vi "ExtractScleraPlane.vi"(11 "Image In":T1) -> (3 "Image Out":T1)   [LabVIEW 2014]
uses:
  <vilib>/vision/Image Controls.llb/IMAQ Image.ctl
  <vilib>/vision/NI_Vision_Development_Module.lvlib
panel:
  out "error out":errorcluster
  in  "error in":errorcluster
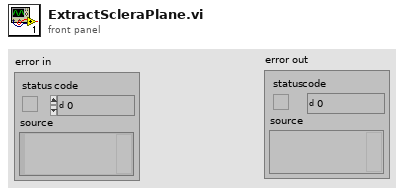
[diagram p1: front panel]
types:
  T1 = typedef "IMAQ Image.ctl" = refnum<image>
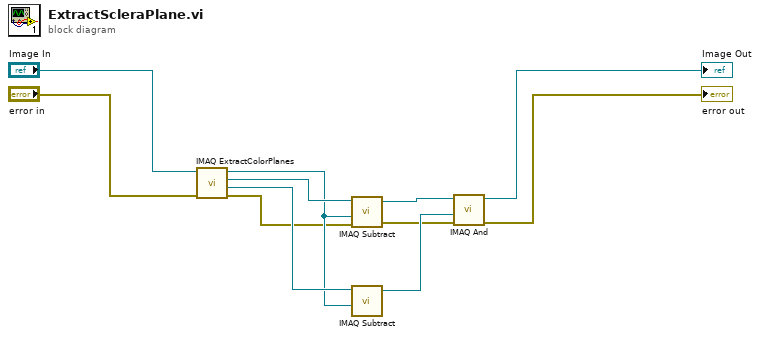
[diagram p0: block diagram]
diagram:
  n1 = call "IMAQ ExtractColorPlanes"("error in (no error)"="error in", "Image Src"="Image In") -> ("error out"=w3:errorcluster, "Blue or Luma or Val or Inten Plane out"=w8:T1, "Green or Sat Plane out"=w9:T1, "Red or Hue Plane out"=w7:T1)  [unwired: 6 in]
  n2 = call "IMAQ Subtract"("Image Src A"=w9, "Image Src B"=w7, "error in (no error)"=w3) -> ("Image Dst Out"=w6:T1, "error out"=w2:errorcluster)  [unwired: 4 in]
  n3 = call "IMAQ Subtract"("Image Src A"=w8, "Image Src B"=w7) -> ("Image Dst Out"=w5:T1)  [unwired: 5 in, 1 out]
  n4 = call "IMAQ And"("error in (no error)"=w2, "Image Src B"=w5, "Image Src A"=w6) -> ("error out"=→"error out":errorcluster, "Image Dst Out"=→"Image Out":T1)  [unwired: 7 in]
